vi "EXPRES Format Shutter Status Message.vi"(8 "error in":errorcluster, 10 "Shutter":T1) -> (0 "error out":errorcluster, 2 "JSON string":string)   [LabVIEW 2016]
uses:
  Controls/Shutter Data.ctl
  Controls/Shutter States.ctl
  Controls/Shutter Status Message.ctl
  Libs/Messages.lvlib
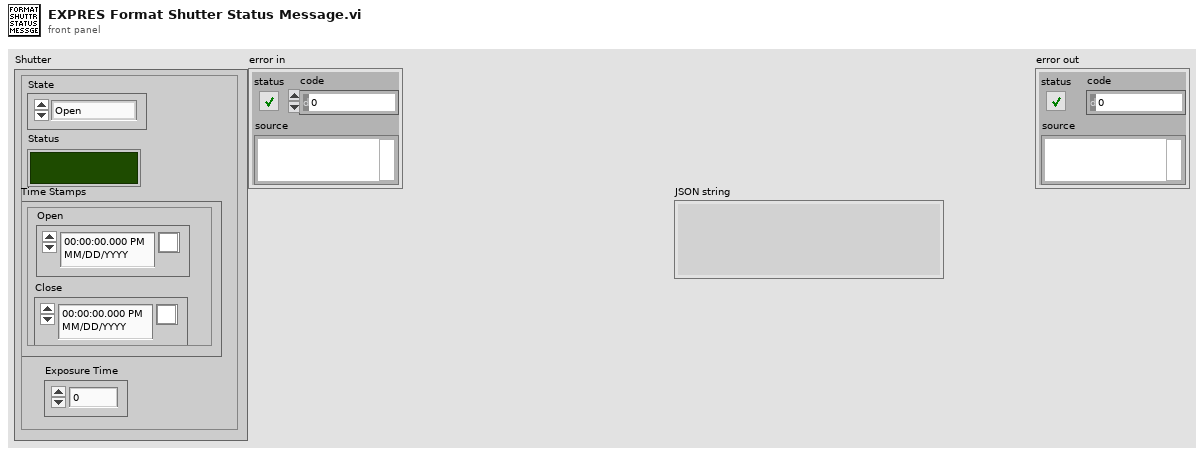
[diagram p1: front panel]
types:
  T1 = typedef "Shutter Data.ctl" = cluster{"Status":bool, "State":T2, "Time Stamps":cluster{"Open":timestamp, "Close":timestamp}, "Exposure Time":dbl}
  T2 = typedef "Shutter States.ctl" = enum16{"Open", "Close", "Wait", "Off", "Arm", "Idle"}
  T3 = typedef "Messages.lvlib/Shutter Status Message.ctl" = cluster{"status":string, "state":string, "exposure":string, "time_opened":string, "time_closed":string}
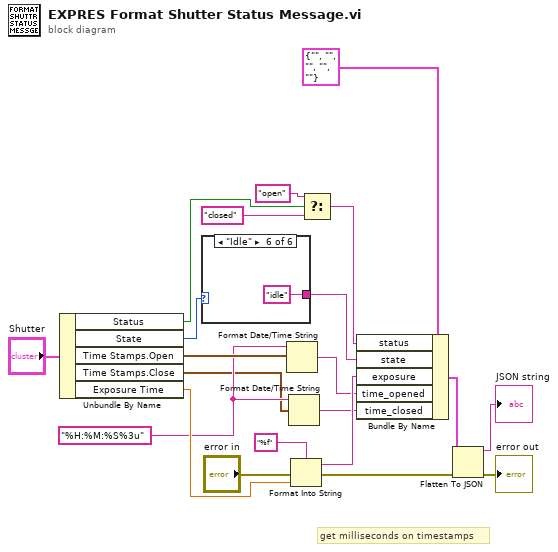
[diagram p0: block diagram]
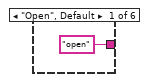
[diagram p2: hidden frame]
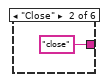
[diagram p3: hidden frame]
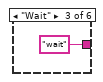
[diagram p4: hidden frame]
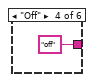
[diagram p5: hidden frame]
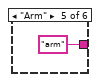
[diagram p6: hidden frame]
diagram:
  w4 = "%H:%M:%S%3u" ("time format string (%c)")
  # "get milliseconds on timestamps"
  n1 = Unbundle By Name("Shutter") -> ("Status"=w20:bool, "State"=w17:T2, "Time Stamps.Open"=w5:timestamp, "Time Stamps.Close"=w2:timestamp, "Exposure Time"=w16:dbl)
  n2 = case shown="\"Idle\"" w17 {
    tunnel: ["open" "close" "wait" "off" "arm" "idle"] -> w12
    frame "Open", Default {
    }
    frame "Close" {
    }
    frame "Wait" {
    }
    frame "Off" {
    }
    frame "Arm" {
    }
    frame "Idle" {
    }
  }
  n3 = Format Date/Time String(time format string (%c)=w4, seconds (now)=w5) -> (date/time string=w3:string)  [unwired: 1 in]
  n4 = Format Date/Time String(time format string (%c)=w4, seconds (now)=w2) -> (date/time string=w1:string)  [unwired: 1 in]
  n5 = Format Into String(format string="%f", error in="error in", w16) -> (resulting string=w11:string, error out=w8:errorcluster)  [unwired: 1 in]
  n6 = Select(t="open", s=w20, f="closed") -> (s? t:f=w13:string)
  n7 = Bundle By Name(cluster=T3 {"status"="", "state"="", "exposure"="", "time_opened"="", "time_closed"=""}, "status"=w13, "state"=w12, "exposure"=w11, "time_opened"=w3, "time_closed"=w1) -> (w10:T3)
  n8 = Flatten To JSON(anything=w10, error in (no error)=w8) -> (JSON string=→"JSON string":string, 11:→"error out":errorcluster)  [unwired: 1 in]
